vi "Read First Frame_.vi"(8 "error in (no error)":errorcluster, 11 "Video File in":refnum<class "Video File.lvclass">) -> (0 "error out":errorcluster, 2 "First Frame?":bool=TRUE, 3 "Video File out":refnum<class "Video File.lvclass">)   [LabVIEW 2018, in "Video File.lvclass"]
uses:
  Video File.lvclass
  Video File.lvclass/Video File.ctl
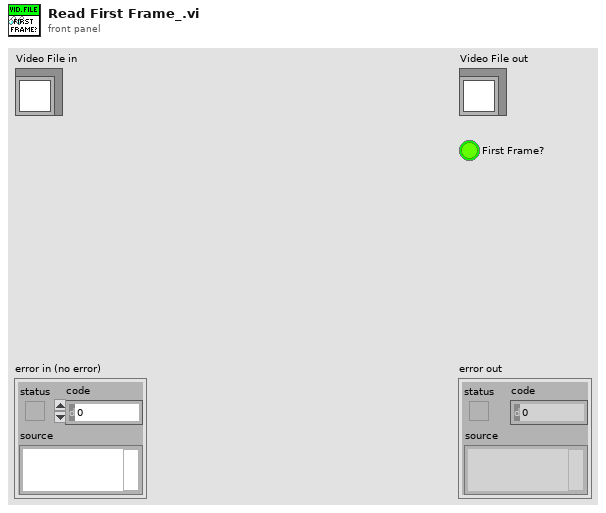
[diagram p1: front panel]
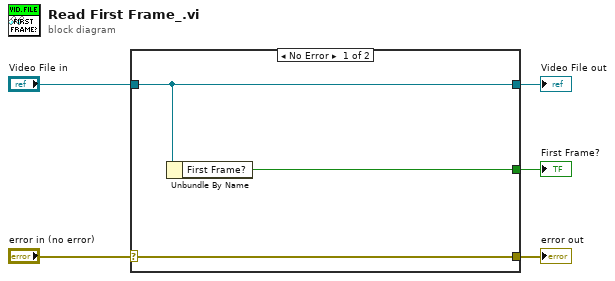
[diagram p0: block diagram]
diagram:
  n1 = case shown="No Error" "error in (no error)" {
    selector: "error in (no error)" -> [w8 w9]
    tunnel: [w8 w9] -> w4
    tunnel: [w7 w10] -> w2
    tunnel: "Video File in" -> [w7 w10]
    tunnel: [w6 _] -> w1
    frame No Error {
      n2 = Unbundle By Name(w7) -> ("First Frame?"=w6:bool)
    }
    frame Error {
    }
  }
  "error out" <- w4
  "Video File out" <- w2
  "First Frame?" <- w1
